vi "fuzzyex Simulate Car position.vi"(4 "Direction":bool, 6 "Steering Angle (Phi)":dbl format="%.2f", 7 "Current Vehicle Orientation (Beta)":dbl format="%.2f", 8 "Current Position Y":dbl format="%.2f", 9 "Current Position X":dbl format="%.2f") -> (1 "New Vehicle Orientation Beta":dbl format="%.2f", 2 "New position Y":dbl format="%.2f", 3 "New position X":dbl format="%.2f")   [LabVIEW 2023]
doc: "This VI is used within the vehicle drive control model to calculate the new vehicle position (Vehicle Center Coordinates X(VC) and Y(VC)) and the vehicle orientation (Beta) for a given steering angle (Phi) and moving direction (Dir := Forward | Backward)."
panel:
  # "Moving Direction (Off=Backward)"
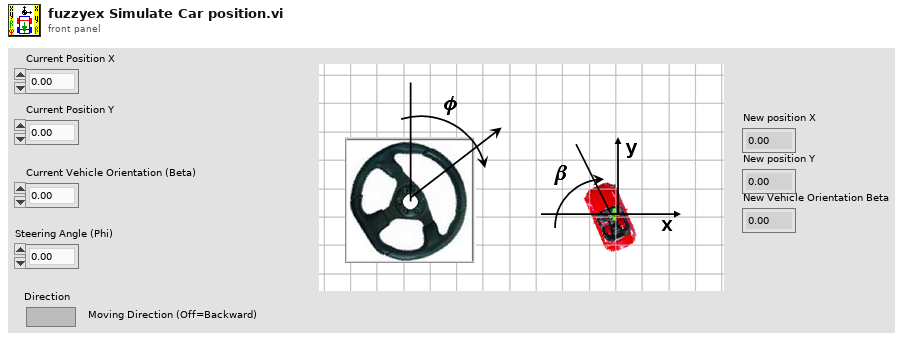
[diagram p1: front panel]
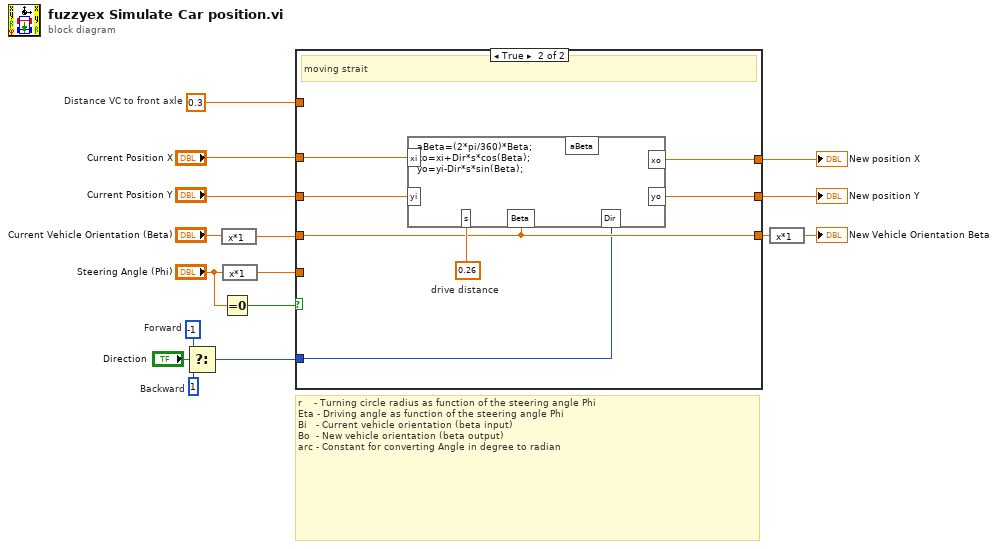
[diagram p0: block diagram]
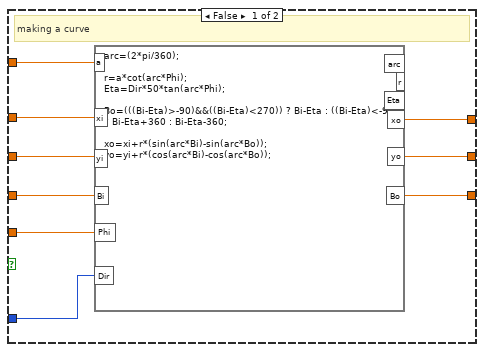
[diagram p2: hidden frame]
diagram:
  w1 = 0.3  # Distance VC to front axle
  w9 = -1  # Forward
  w8 = 1  # Backward
  # "r    - Turning circle radius as function of the steering angle Phi\nEta - Driving angle as function of the steering angle Phi\nBi   - Current vehicle orientation (beta input)\nBo  - New vehicle orientation (beta output)\narc - Constant for converting Angle in degree to radian"
  n1 = Select(t=w9, s="Direction", f=w8) -> (s? t:f=w7:i32)
  n2 = expression code="x*1"("Current Vehicle Orientation (Beta)") -> (w5:dbl)
  n3 = Equal To 0?(x="Steering Angle (Phi)") -> (x = 0?=w16:bool)
  n4 = expression code="x*1"("Steering Angle (Phi)") -> (w6:dbl)
  n5 = case shown="True" w16 {
    tunnel: w5 -> [w23 w31]
    tunnel: [w21 w31] -> w3
    tunnel: "Current Position X" -> [w25 w30]
    tunnel: "Current Position Y" -> [w24 w29]
    tunnel: [w20 w28] -> w13
    tunnel: [w22 w27] -> w12
    tunnel: w6 -> [w19 _]
    tunnel: w7 -> [w18 w26]
    tunnel: w1 -> [w17 _]
    frame False {
      # "making a curve"
      n6 = formula code="arc=(2*pi/360);\n\nr=a*cot(arc*Phi);\nEta=Dir*50*tan(arc*Phi);\n\nBo=(((Bi-Eta)>-90)&&((Bi-Eta)<270)) ? Bi-Eta : ((Bi-Eta)<-90) ? Bi-Eta+360 : Bi-Eta-360;\n\nxo=xi+r*(sin(arc*Bi)-sin(arc*Bo));\nyo=yi+r*(cos(arc*Bi)-cos(arc*Bo));"("xi"=w25, "yi"=w24, "Bi"=w23, "Phi"=w19, "a"=w17, "Dir"=w18) -> ("yo"=w22:dbl, "Bo"=w21:dbl, "xo"=w20:dbl)  [unwired: 3 out]
    }
    frame True {
      w32 = 0.26  # drive distance
      # "moving strait"
      n7 = formula code="aBeta=(2*pi/360)*Beta;\nxo=xi+Dir*s*cos(Beta);\nyo=yi-Dir*s*sin(Beta);"("xi"=w30, "yi"=w29, "s"=w32, "Beta"=w31, "Dir"=w26) -> ("xo"=w28:dbl, "yo"=w27:dbl)  [unwired: 1 out]
    }
  }
  "New position X" <- w13
  "New position Y" <- w12
  n8 = expression code="x*1"(w3) -> (→"New Vehicle Orientation Beta":dbl)
